vi "Caption Set Fuel.vi"(0 "Reference Cluster":T1) -> ()   [LabVIEW 2017, in "GUI.lvlib"]
uses:
  GUI.lvlib
  Konfiguracja/Konfiguracja.lvlib
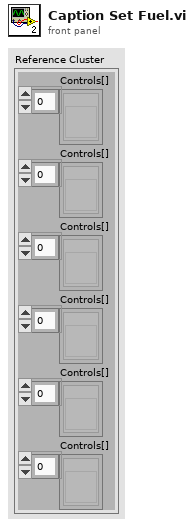
[diagram p1: front panel]
types:
  T1 = cluster{"Controls[]":refnum<vi>[], "Controls[]":refnum<vi>[], "Controls[]":refnum<vi>[], "Controls[]":refnum<vi>[], "Controls[]":refnum<vi>[], "Controls[]":refnum<vi>[]}
  T2 = cluster{"Paliwo 1":string, "Paliwo 2":string, "Paliwo 3":string, "Paliwo 4":string, "Paliwo 5":string, "Paliwo 6":string}
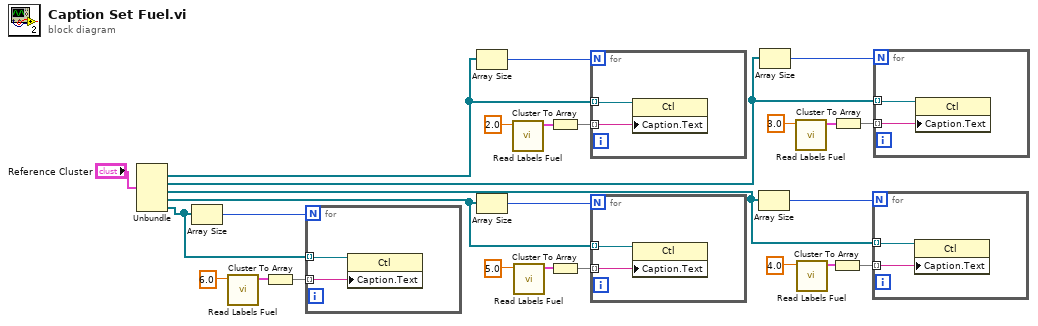
[diagram p0: block diagram]
diagram:
  n1 = Unbundle("Reference Cluster") -> ("Controls[]"=w23:refnum<vi>[], "Controls[]"=w20:refnum<vi>[], "Controls[]"=w17:refnum<vi>[], "Controls[]"=w14:refnum<vi>[], "Controls[]"=w11:refnum<vi>[])  [unwired: 1 out]
  n2 = Array Size(array=w11) -> (size(s)=w13:i32)
  n3 = call "Read Labels Fuel.vi"("Slave ID"=6.0) -> ("Etykiety P1-6"=w2:T2)  [unwired: 10 in]
  n4 = Cluster To Array(cluster=w2) -> (array=w12:string[])
  n5 = for {
    N: w13 -> [_]
    tunnel: w11 -> [w28] mode=indexing
    tunnel: w12 -> [w27] mode=indexing
    n6 = property class="Ctl"(reference=w28, "Caption.Text"=w27) -> ()  [unwired: 1 in, 2 out]
  }
  n7 = Array Size(array=w23) -> (size(s)=w25:i32)
  n8 = Array Size(array=w14) -> (size(s)=w16:i32)
  n9 = call "Read Labels Fuel.vi"("Slave ID"=2.0) -> ("Etykiety P1-6"=w10:T2)  [unwired: 10 in]
  n10 = call "Read Labels Fuel.vi"("Slave ID"=5.0) -> ("Etykiety P1-6"=w4:T2)  [unwired: 10 in]
  n11 = Cluster To Array(cluster=w10) -> (array=w24:string[])
  n12 = Cluster To Array(cluster=w4) -> (array=w15:string[])
  n13 = for {
    N: w25 -> [_]
    tunnel: w23 -> [w30] mode=indexing
    tunnel: w24 -> [w29] mode=indexing
    n14 = property class="Ctl"(reference=w30, "Caption.Text"=w29) -> ()  [unwired: 1 in, 2 out]
  }
  n15 = for {
    N: w16 -> [_]
    tunnel: w14 -> [w32] mode=indexing
    tunnel: w15 -> [w31] mode=indexing
    n16 = property class="Ctl"(reference=w32, "Caption.Text"=w31) -> ()  [unwired: 1 in, 2 out]
  }
  n17 = Array Size(array=w17) -> (size(s)=w19:i32)
  n18 = Array Size(array=w20) -> (size(s)=w22:i32)
  n19 = call "Read Labels Fuel.vi"("Slave ID"=3.0) -> ("Etykiety P1-6"=w8:T2)  [unwired: 10 in]
  n20 = call "Read Labels Fuel.vi"("Slave ID"=4.0) -> ("Etykiety P1-6"=w6:T2)  [unwired: 10 in]
  n21 = Cluster To Array(cluster=w6) -> (array=w18:string[])
  n22 = Cluster To Array(cluster=w8) -> (array=w21:string[])
  n23 = for {
    N: w19 -> [_]
    tunnel: w17 -> [w34] mode=indexing
    tunnel: w18 -> [w33] mode=indexing
    n24 = property class="Ctl"(reference=w34, "Caption.Text"=w33) -> ()  [unwired: 1 in, 2 out]
  }
  n25 = for {
    N: w22 -> [_]
    tunnel: w20 -> [w36] mode=indexing
    tunnel: w21 -> [w35] mode=indexing
    n26 = property class="Ctl"(reference=w36, "Caption.Text"=w35) -> ()  [unwired: 1 in, 2 out]
  }
